vi "TCP Query.vi"(8 "error in":errorcluster) -> (0 "error out":errorcluster, 3 "Busy?":bool)   [LabVIEW 2013]
panel:
  out "data out":string
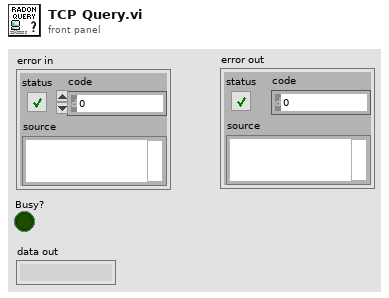
[diagram p1: front panel]
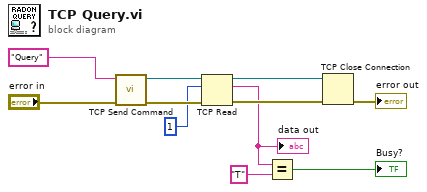
[diagram p0: block diagram]
diagram:
  n1 = call "TCP Send Command.vi"("error in"="error in", "Command"="Query") -> ("error out"=w9:errorcluster, "connection ID out"=w8:refnum<k5>)  [unwired: 8 in]
  n2 = TCP Read(connection ID=w8, bytes to read=1, error in (no error)=w9) -> (connection ID out=w5:refnum<k5>, data out=w3:string, error out=w6:errorcluster)  [unwired: 2 in]
  "data out" <- w3
  n3 = Equal?(x=w3, y="T") -> (x = y?=→"Busy?":bool)
  n4 = TCP Close Connection(connection ID=w5, error in (no error)=w6) -> (error out=→"error out":errorcluster)  [unwired: 1 in, 1 out]
